vi "Remove_IconEd_Data.vi"(8 "error in (no error)":errorcluster, 10 "saveLevel":u32, 11 "Build in":refnum<class "AB_Build.lvclass">) -> (0 "error out":errorcluster, 2 "remove":bool, 3 "Build out":refnum<class "AB_Build.lvclass">)   [LabVIEW 2020, in "AB_Build.lvclass"]
uses:
  <vilib>/AppBuilder/AB_Classes/Build/AB_Build.lvclass
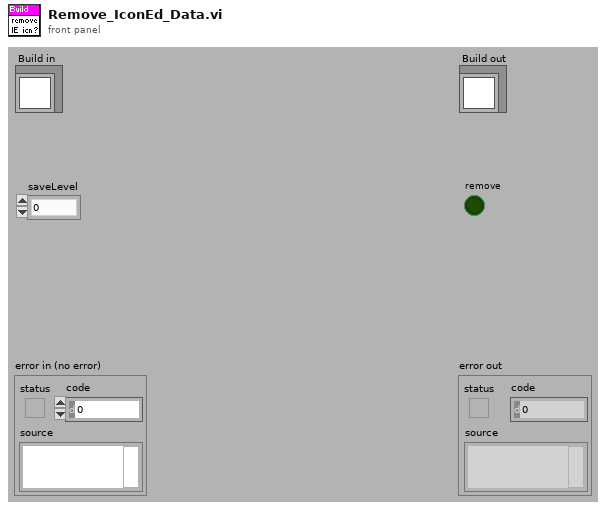
[diagram p1: front panel]
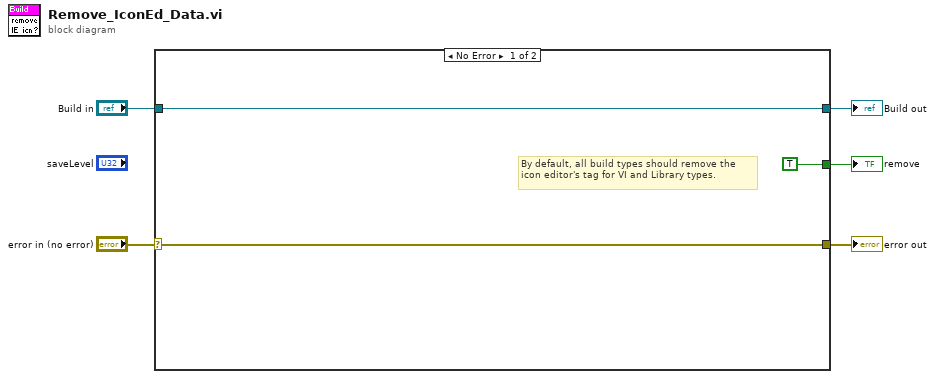
[diagram p0: block diagram]
diagram:
  n1 = case shown="No Error" "error in (no error)" {
    selector: "error in (no error)" -> [w8 w10]
    tunnel: [w8 w10] -> w4
    tunnel: [w7 w9] -> w2
    tunnel: "Build in" -> [w7 w9]
    tunnel: [TRUE _] -> w1
    frame No Error {
      # "By default, all build types should remove the icon editor's tag for VI and Library types."
    }
    frame Error {
    }
  }
  "error out" <- w4
  "Build out" <- w2
  "remove" <- w1
